vi "SPI_Write_CTRL4.vi"(1 "bit_index":i32, 3 "rising_edge":bool) -> ()   [LabVIEW 2019]
doc: "This Vi Read a slave message based on SPI protocol. It works with a clock handler and inside a loop"
uses:
  <vilib>/rvi/eio/common/nirviEmuTemplateMethod_errors.vi
  <vilib>/eio/EIONode/EIONode.xnode
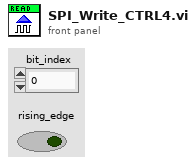
[diagram p1: front panel]
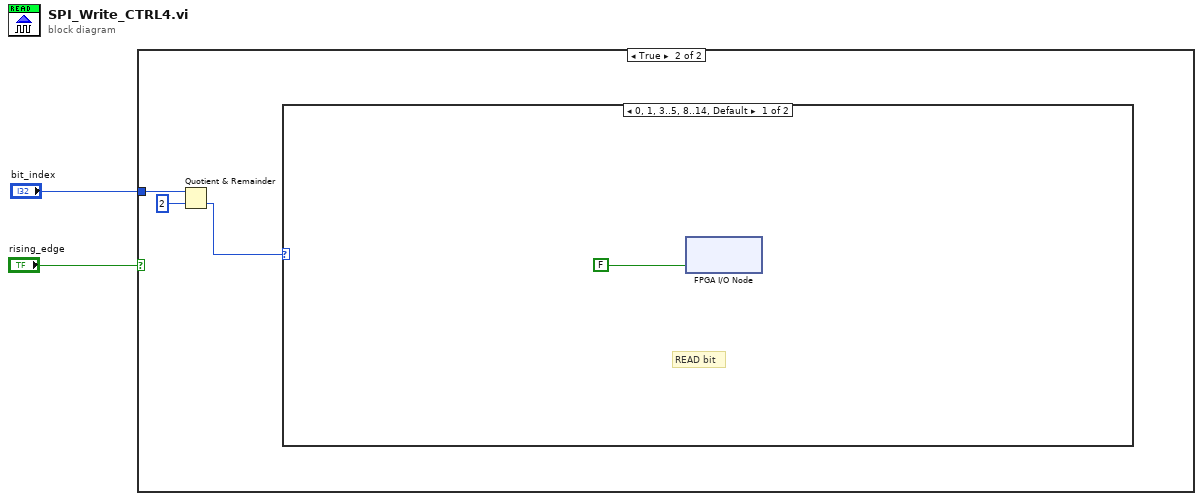
[diagram p0: block diagram]
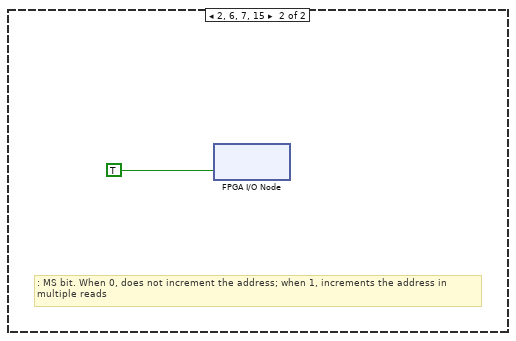
[diagram p3: hidden frame]
diagram:
  n1 = case shown="True" "rising_edge" {
    tunnel: "bit_index" -> [_ w5]
    frame False {
    }
    frame True {
      n2 = Quotient & Remainder(x=w5, y=2) -> (floor(x/y)=w3:i32)  [unwired: 1 out]
      n3 = case shown="0, 1, 3..5, 8..14, Default" w3 {
        frame 0, 1, 3..5, 8..14, Default {
          # "READ bit"
          n4 = xnode "FPGA I/O Node"("SDI"=FALSE) -> ()  [unwired: 1 in, 1 out]
        }
        frame 2, 6, 7, 15 {
          # ": MS bit. When 0, does not increment the address; when 1, increments the address in\nmultiple reads"
          n5 = xnode "FPGA I/O Node"("SDI"=TRUE) -> ()  [unwired: 1 in, 1 out]
        }
      }
    }
  }
